vi "From Bytes.vi"(8 "error in (no error)":errorcluster, 10 "Bytes":u8[](array[numeric])) -> (0 "error out":errorcluster, 3 "UUID out":refnum<class "UUID.lvclass">)   [LabVIEW 2015, in "UUID.lvclass"]
uses:
  UUID.lvclass
  UUID.lvclass/UUID.ctl
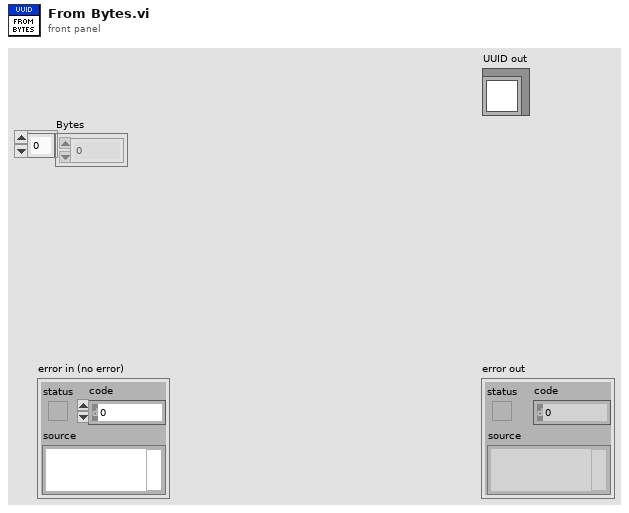
[diagram p1: front panel]
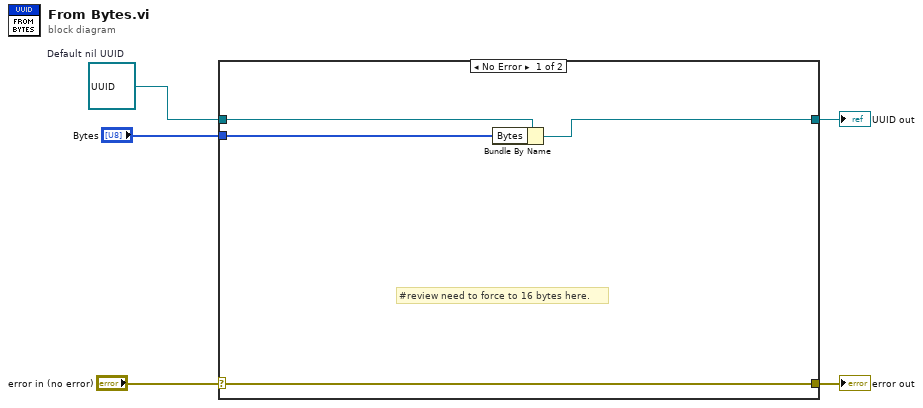
[diagram p0: block diagram]
diagram:
  w3 = refnum<class "UUID.lvclass"> refnum  # Default nil UUID
  n1 = case shown="No Error" "error in (no error)" {
    selector: "error in (no error)" -> [w8 w11]
    tunnel: [w8 w11] -> w4
    tunnel: [w7 w10] -> w2
    tunnel: w3 -> [w9 w10]
    tunnel: "Bytes" -> [w6 _]
    frame No Error {
      # "#review need to force to 16 bytes here."
      n2 = Bundle By Name(cluster=w9, "Bytes"=w6) -> (w7:refnum<class "UUID.lvclass">)
    }
    frame Error {
    }
  }
  "error out" <- w4
  "UUID out" <- w2
